vi "Setup Pressure Transducers (SubVI).vi"(0 "Refnum in":refnum<k21>, 5 "Cluster Out":T1(array[cluster]), 9 "Error In":errorcluster) -> (3 "Units":string[](array[string]), 4 "Refnum out":refnum<k21>, 6 "# PT":i32, 8 "Max Out":dbl[](array[numeric]), 10 "Array":string[](array[string]), 12 "PT Units Num":dbl[](array[numeric]), 13 "Min Out":dbl[](array[numeric]), 14 "# Pressure Transducers":i32, 15 "Error Out":errorcluster)   [LabVIEW 2011]
uses:
  <vilib>/Utility/error.llb/DialogType.ctl
  <vilib>/DAQmx/create/channels.llb/DAQmx Create Channel (AI-Voltage-Basic).vi
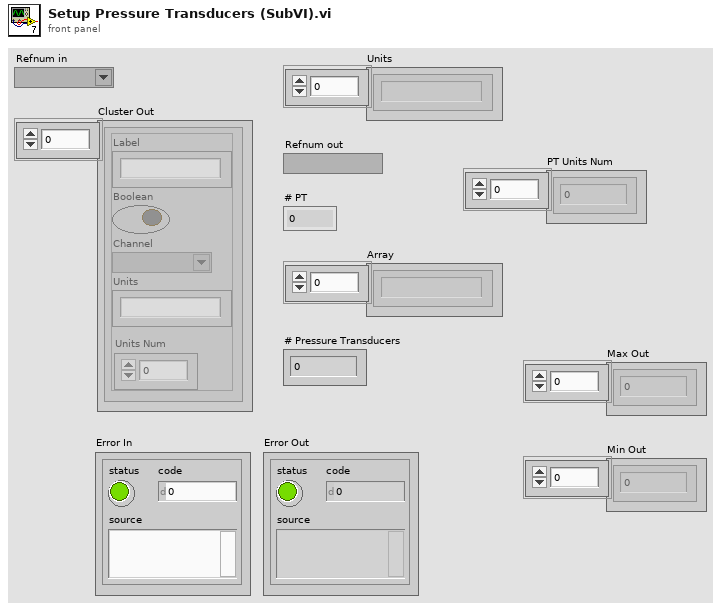
[diagram p1: front panel]
types:
  T1 = cluster{"Label":string, "Boolean":bool, "Channel":tag, "Units":string, "Units Num":dbl}[]
  T2 = typedef "DialogType.ctl" = u16
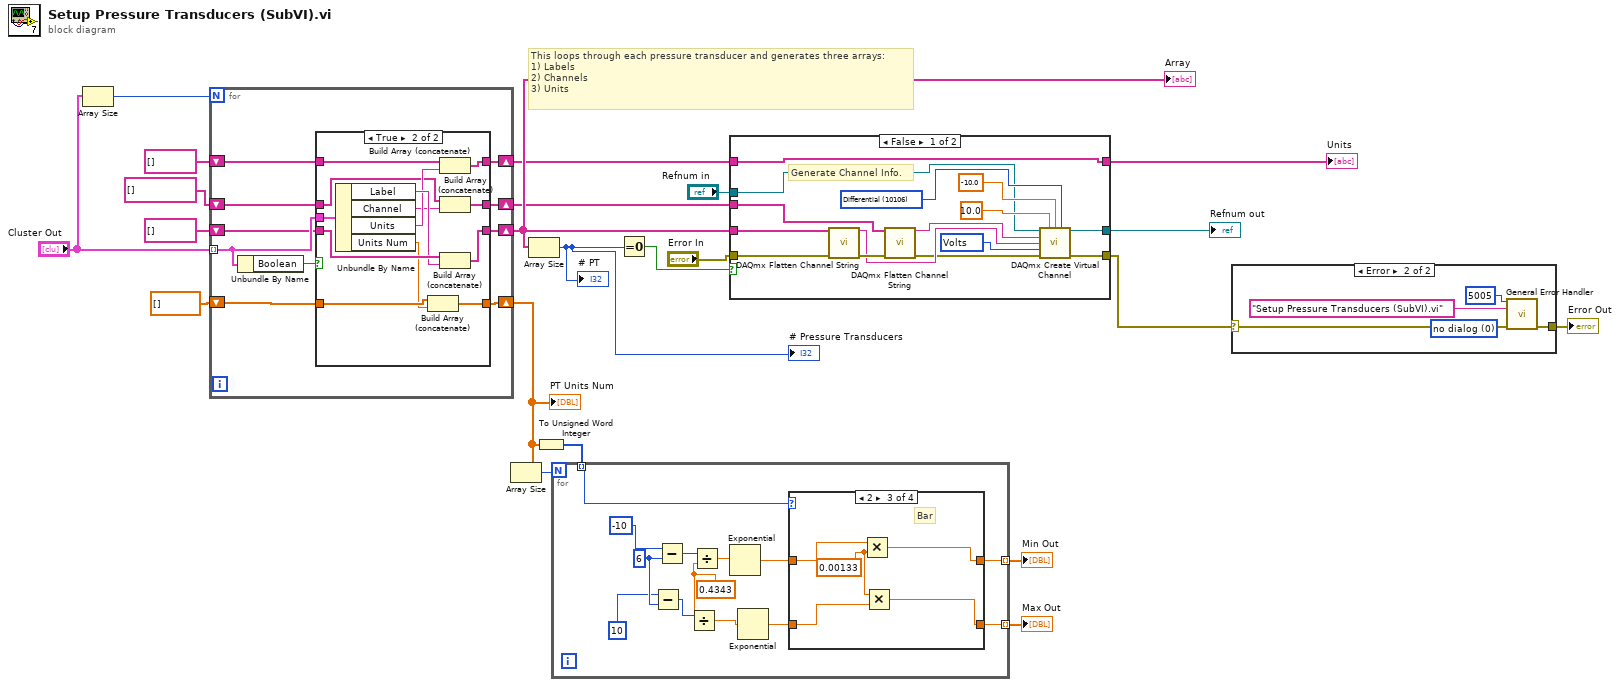
[diagram p0: block diagram]
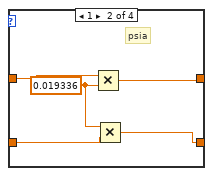
[diagram p4: hidden frame]
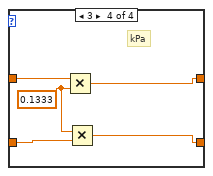
[diagram p5: hidden frame]
diagram:
  # "This loops through each pressure transducer and generates three arrays: \n1) Labels\n2) Channels\n3) Units"
  n1 = Array Size(array="Cluster Out") -> (size(s)=w10:i32)
  n2 = for {
    N: w10 -> [_]
    tunnel: "Cluster Out" -> [w31] mode=indexing
    shift-right: [w30] -> w21
    shift-left: string[] [] -> [w29]
    shift-right: [w28] -> w17
    shift-left: string[] [] -> [w27]
    shift-right: [w26] -> w16
    shift-left: tag[] [] -> [w25]
    shift-right: [w24] -> w7
    shift-left: dbl[] [] -> [w23]
    n3 = Unbundle By Name(w31) -> ("Boolean"=w32:bool)
    n4 = case shown="True" w32 {
      tunnel: w31 -> [_ w49]
      tunnel: [w36 w48] -> w30
      tunnel: w29 -> [w36 w47]
      tunnel: [w34 w44] -> w28
      tunnel: w27 -> [w34 w43]
      tunnel: [w35 w41] -> w26
      tunnel: w25 -> [w35 w40]
      tunnel: [w33 w39] -> w24
      tunnel: w23 -> [w33 w38]
      frame False {
      }
      frame True {
        n5 = Unbundle By Name(w49) -> ("Label"=w46:string, "Channel"=w42:tag, "Units"=w45:string, "Units Num"=w37:dbl)
        n6 = Build Array (concatenate)(w38, w37) -> (w39:dbl[])
        n7 = Build Array (concatenate)(w43, w45) -> (w44:string[])
        n8 = Build Array (concatenate)(w40, w42) -> (w41:tag[])
        n9 = Build Array (concatenate)(w47, w46) -> (w48:string[])
      }
    }
  }
  "Array" <- w21
  "PT Units Num" <- w7
  n10 = Array Size(array=w7) -> (size(s)=w5:i32)
  n11 = Array Size(array=w21) -> (size(s)=w22:i32)
  "# PT" <- w22
  "# Pressure Transducers" <- w22
  n12 = To Unsigned Word Integer(number=w7) -> (unsigned 16bit integer=w6:u16[])
  n13 = for {
    N: w5 -> [_]
    tunnel: w6 -> [w62] mode=indexing
    tunnel: [w51] -> w3 mode=indexing
    tunnel: [w50] -> w4 mode=indexing
    w58 = 0.4343
    w61 = 6 ("y")
    n14 = Subtract(x=10, y=w61) -> (x-y=w59:i32)
    n15 = Subtract(x=-10, y=w61) -> (x-y=w60:i32)
    n16 = Divide(x=w59, y=w58) -> (x/y=w56:dbl)
    n17 = Divide(x=w60, y=w58) -> (x/y=w57:dbl)
    n18 = Exponential(1:w57) -> (0:w53:dbl)
    n19 = Exponential(1:w56) -> (0:w52:dbl)
    n20 = case shown="2" w62 {
      tunnel: w53 -> [w64 w69 w71 w76]
      tunnel: w52 -> [w63 w68 w72 w77]
      tunnel: [w64 w66 w74 w79] -> w51
      tunnel: [w63 w67 w73 w78] -> w50
      frame 0, Default {
        # "Torr"
      }
      frame 1 {
        w65 = 0.019336 ("y")
        # "psia"
        n21 = Multiply(x=w69, y=w65) -> (x*y=w66:dbl)
        n22 = Multiply(x=w65, y=w68) -> (x*y=w67:dbl)
      }
      frame 2 {
        w70 = 0.00133 ("y")
        # "Bar"
        n23 = Multiply(x=w71, y=w70) -> (x*y=w74:dbl)
        n24 = Multiply(x=w70, y=w72) -> (x*y=w73:dbl)
      }
      frame 3 {
        w75 = 0.1333 ("y")
        # "kPa"
        n25 = Multiply(x=w76, y=w75) -> (x*y=w79:dbl)
        n26 = Multiply(x=w75, y=w77) -> (x*y=w78:dbl)
      }
    }
  }
  "Max Out" <- w4
  "Min Out" <- w3
  n27 = Equal To 0?(x=w22) -> (x = 0?=w15:bool)
  n28 = case shown="False" w15 {
    tunnel: w21 -> [w94 _]
    tunnel: w16 -> [w91 _]
    tunnel: w17 -> [w80 w95]
    tunnel: "Error In" -> [w93 w96]
    tunnel: "Refnum in" -> [w83 w97]
    tunnel: [w82 w97] -> w19
    tunnel: [w81 w96] -> w2
    tunnel: [w80 w95] -> w20
    frame False {
      w84 = 10106 items=["default"=-1, "RSE"=10083, "NRSE"=10078, "Differential"=10106, "Pseudodifferential"=12529] ("input terminal configuration")
      w88 = 10348 items=["Volts"=10348, "From Custom Scale"=10065] ("units")
      # "Generate Channel Info."
      n29 = call <vilib>:"DAQmx Flatten Channel String.vi"("names in"=w94, "error in"=w93) -> ("names out"=w90:string, "error out"=w92:errorcluster)  [unwired: 12 in]
      n30 = call <vilib>:"DAQmx Flatten Channel String.vi"("names in"=w91, "error in"=w92) -> ("names out"=w89:string, "error out"=w87:errorcluster)  [unwired: 12 in]
      n31 = call-poly <vilib>:"DAQmx Create Virtual Channel.vi"("task in"=w83, "maximum value"=10.0, "minimum value"=-10.0, "input terminal configuration"=w84, "physical channels"=w89, "name to assign"=w90, "units"=w88, "error in"=w87) -> ("task out"=w82:refnum<k21>, "error out"=w81:errorcluster)  [unwired: 6 in]
    }
    frame True {
      # "Zero elements: Skip"
    }
  }
  "Units" <- w20
  "Refnum out" <- w19
  n32 = case shown="Error" w2 {
    selector: w2 -> [w98 w103]
    tunnel: [w98 w102] -> w1
    frame No Error {
    }
    frame Error {
      w99 = T2 0 items=["no dialog", "OK message", "continue or stop message", "OK message + warnings", "continue/stop + warnings"] ("type of dialog (OK msg:1)")
      n33 = call <vilib>:"General Error Handler.vi"("[error code] (0)"=5005, "[error source] (\" \")"="Setup Pressure Transducers (SubVI).vi" ("[error source] (\" \")"), "type of dialog (OK msg:1)"=w99, "error in (no error)"=w103) -> ("error out"=w102:errorcluster)  [unwired: 7 in, 4 out]
    }
  }
  "Error Out" <- w1
